vi "Actor Core.vi"(8 "error in":errorcluster, 11 "CS++OPCUAInterface in":refnum<class "CS++OPCUAInterface.lvclass">) -> (0 "error out":errorcluster, 3 "Actor out":refnum<class "Actor.lvclass">)   [LabVIEW 2015, in "CS++OPCUAInterface.lvlib" / "CS++OPCUAInterface.lvclass"]
doc: "Register OPCUA-Item vor values change events and write new data to PV-Read-URLs.\n\n\n(<B>Filename</B>: Actor Framework.lvlib:Actor.lvclass:Actor Core.vi)\n\nReceives messages to the actor, reacts to them, and initiates any error handling that may shut the actor down.\n\nDescendant classes may override this VI to append parallel tasks for the actor to complete while it handles messages. Overrides use the Call Parent Method node."
uses:
  CS++OPCUAInterface.lvclass
  <vilib>/ActorFramework/Actor/Actor.lvclass
  CS++OPCUAInterface.lvclass/CS++OPCUAInterface.ctl
  CSPP_Core/Actors/CS++BaseActor/CS++BaseActor.lvclass/CS++BaseActor.ctl
  CSPP_Core/Classes/CS++ProcessVariables/ProcessVariable/PV.lvclass
  CSPP_Core/Classes/CS++ProcessVariables/ProcessVariable/PV.lvclass/PV.ctl
  <vilib>/ActorFramework/Actor/Actor.lvclass/Actor.ctl
  <vilib>/ActorFramework/Message Enqueuer/Message Enqueuer.lvclass/Message Enqueuer.ctl
  <vilib>/ActorFramework/Report Error Msg/Report Error Msg.lvclass/Report Error Msg.ctl
  CSPP_Core/Classes/CS++ProcessVariables/ProcessVariable/Write Data.vi
  CSPP_Core/Classes/CS++ProcessVariables/ProcessVariable/Write Timestamp.vi
  CSPP_Core/Classes/CS++ProcessVariables/ProcessVariable/Write status.vi
  CSPP_Core/Classes/CS++ProcessVariables/ProcessVariable/Write Quality.vi
  CSPP_Core/Classes/CS++ProcessVariables/ProcessVariable/Write Error.vi
  CSPP_Core/Actors/CS++BaseActor/Read Polling Interval.vi
  <vilib>/ActorFramework/Message Enqueuer/Init from Existing Queue.vi
  <vilib>/ActorFramework/Message Enqueuer/Enqueue.vi
  <vilib>/ActorFramework/Message Priority Queue/Priority Enqueue.vi
  <vilib>/ActorFramework/Message Enqueuer/Message Enqueuer.lvclass
  <vilib>/ActorFramework/Report Error Msg/Report Error Msg.lvclass
  CSPP_Core/Actors/CS++BaseActor/CS++BaseActor.lvclass
  <vilib>/OPCUA/NI OPC UA Client.lvlib
  CSPP_Core/Classes/CS++ProcessVariables/PVConnection/PVConnection.lvclass
panel:
  out "Data":T1
  out "Size":i32
  out "OPCUA-Item":string
  out "PV-URL":string
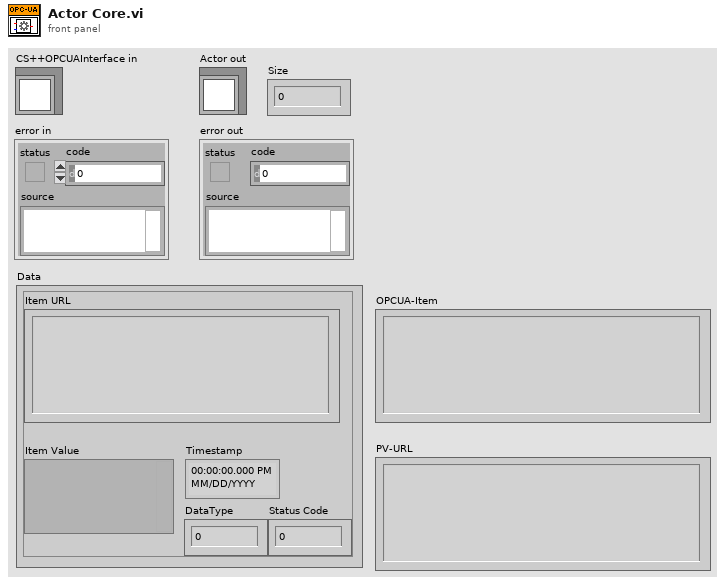
[diagram p1: front panel]
types:
  T1 = cluster{"Item URL":string, "Item Value":variant, "Timestamp":timestamp, "DataType":u32, "Status Code":u32}
  T2 = cluster{"queue size(1)":u32, "discard oldest(T)":bool}
  T3 = cluster{"Item URL":string, "Item Value":variant, "Timestamp":timestamp, "DataType":u32, "status code":u32}[]
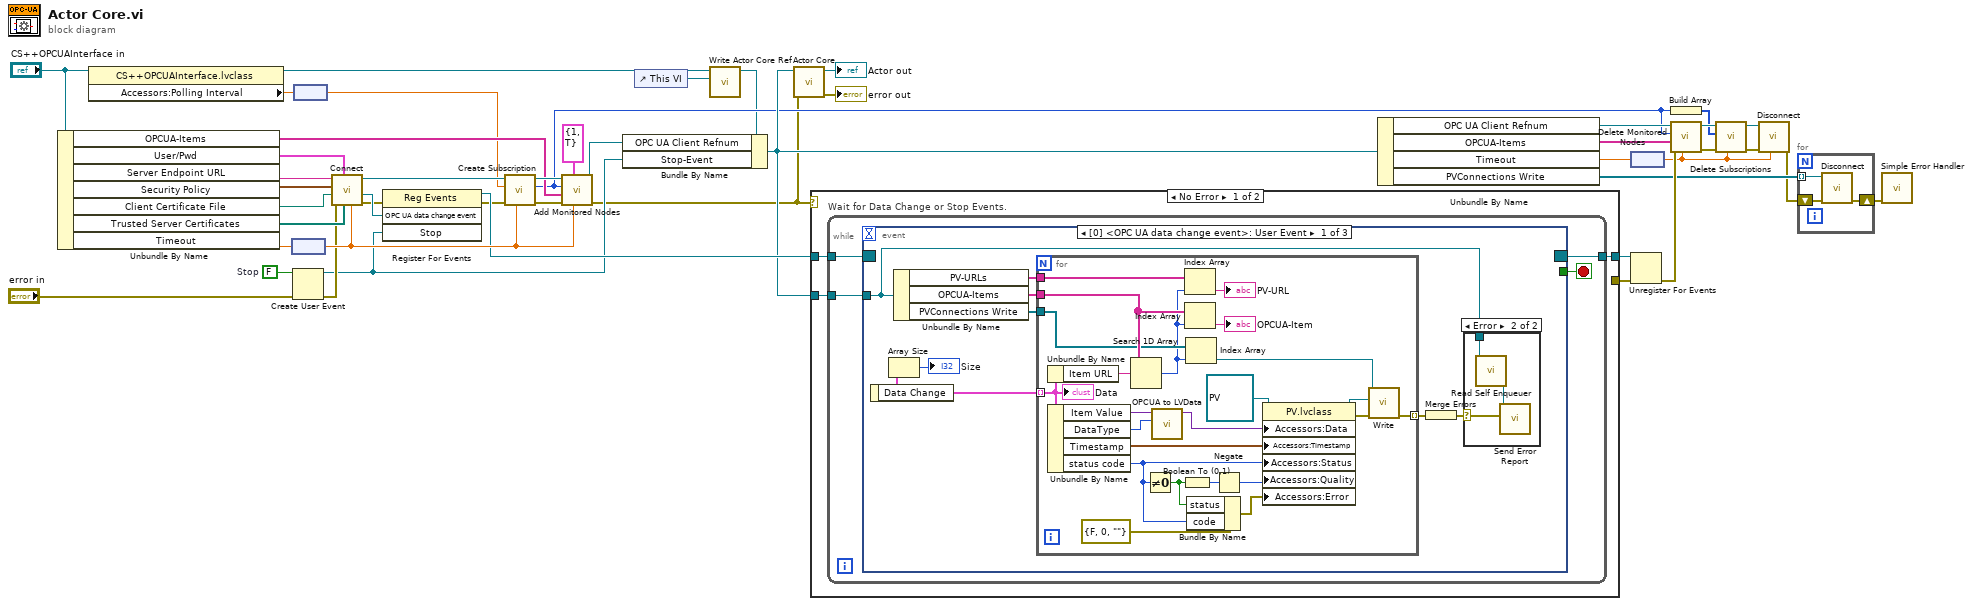
[diagram p0: block diagram]
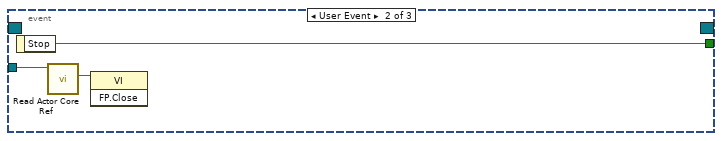
[diagram p3: hidden frame]
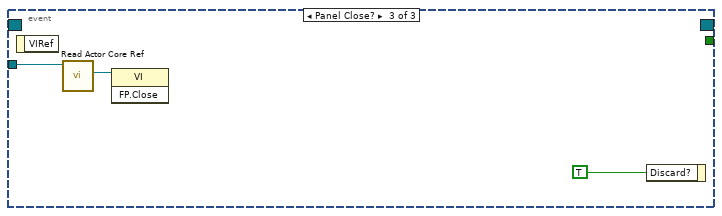
[diagram p4: hidden frame]
diagram:
  w28 = FALSE  # Stop
  n1 = Unbundle By Name("CS++OPCUAInterface in") -> ("OPCUA-Items"=w35:string[], "User/Pwd"=w44:cluster{"Username":string, "Password":string}, "Server Endpoint URL"=w45:string, "Security Policy"=w43:cluster{"Message Mode":u16, "Security":u16}, "Client Certificate File"=w42:path, "Trusted Server Certificates"=w41:path[], "Timeout"=w40:dbl[unit])
  n2 = property class="CS++OPCUAInterface.lvclass"(reference="CS++OPCUAInterface in") -> (reference out=w3:refnum<class "CS++OPCUAInterface.lvclass">, "Accessors:Polling Interval"=w9:dbl[unit])  [unwired: 1 in, 1 out]
  n3 = node(w40) -> (w34:dbl)
  n4 = Create User Event(user event datatype=w28, error in="error in") -> (user event=w25:refnum<user-event>, error out=w26:errorcluster)
  n5 = node(w9) -> (w31:dbl)
  n6 = call <vilib>:"Connect.vi"("timeout (5000 ms)"=w34, "trusted server certificates"=w41, "username/password"=w44, "error in (no error)"=w26, "client certificate file"=w42, "security policy"=w43, "server endpoint URL"=w45) -> ("error out"=w30:errorcluster, "OPC UA data change event"=w39:refnum<user-event>, "OPC UA client refnum out"=w38:refnum<k21>)  [unwired: 2 in]
  n7 = register-events(error in=w30, w39, w25) -> (reference out=w32:refnum<event-registration>, error out=w29:errorcluster)  [unwired: 1 in]
  n8 = call <vilib>:"Create Subscription.vi"("timeout (5000 ms)"=w34, "error in (no error)"=w29, "update rate (1000 ms)"=w31, "OPC UA client refnum in"=w38) -> ("error out"=w36:errorcluster, "subscription ID out"=w17:u32, "OPC UA client refnum out"=w37:refnum<k21>)  [unwired: 5 in]
  n9 = call <vilib>:"Add Monitored Nodes.vi"("timeout (5000 ms)"=w34, "notification queue settings"=T2 {"queue size(1)"=1, "discard oldest(T)"=TRUE}, "error in (no error)"=w36, "array of node path"=w35, "subscription ID in"=w17, "OPC UA client refnum in"=w37) -> ("error out"=w8:errorcluster, "OPC UA client refnum out"=w33:refnum<k21>)  [unwired: 3 in, 1 out]
  n10 = control-ref of="This VI"() -> (w1:refnum<vi>)
  n11 = call "Write Actor Core Ref.vi"("Actor Core Ref"=w1, "CS++BaseActor in"=w3) -> ("CS++BaseActor out"=w2:refnum<class "CS++OPCUAInterface.lvclass">)  [unwired: 8 in, 1 out]
  n12 = Bundle By Name(cluster=w2, "OPC UA Client Refnum"=w33, "Stop-Event"=w25) -> (w20:refnum<class "CS++OPCUAInterface.lvclass">)
  n13 = call-parent "Actor Core.vi"("error in"=w8, "CS++BaseActor in"=w20) -> ("error out"=→"error out":errorcluster, "Actor out"=→"Actor out":refnum<class "Actor.lvclass">)  [unwired: 8 in]
  n14 = case shown="No Error" w8 {
    selector: w8 -> [_ w95]
    tunnel: w32 -> [w50 w96]
    tunnel: [w49 w96] -> w24
    tunnel: w20 -> [w48 _]
    tunnel: [_ w95] -> w7
    frame No Error {
      n15 = while "Wait for Data Change or Stop Events." {
        tunnel: w50 -> [w54]
        tunnel: w48 -> [w51]
        tunnel: [w52] -> w49
        stop <- w53 stop-if-true
        n16 = event shown="[0] <OPC UA data change event>: User Event" {
          selector: w54 -> [_ _ _]
          dyn-events: [_ _ _] -> w52
          timeout: _ -> [_ _ _]
          tunnel: [_ w91 _] -> w53
          tunnel: w51 -> [w56 w90 w92]
          event User Event {
            n17 = event-data() -> ("Data Change"=w59:T3)  [unwired: 1 in]
            n18 = Array Size(array=w59) -> (size(s)=→"Size":i32)
            n19 = Unbundle By Name(w56) -> ("PV-URLs"=w62:string[], "OPCUA-Items"=w61:string[], "PVConnections Write"=w58:refnum<class "PVConnection.lvclass">[])
            n20 = for {
              tunnel: w62 -> [w88]
              tunnel: w61 -> [w85]
              tunnel: w59 -> [w81] mode=indexing
              tunnel: w58 -> [w83]
              tunnel: [w71] -> w57 mode=indexing
              n21 = Unbundle By Name(w81) -> ("Item URL"=w84:string)
              n22 = Unbundle By Name(w81) -> ("Item Value"=w68:variant, "DataType"=w66:u32, "Timestamp"=w80:timestamp, "status code"=w75:u32)
              n23 = Search 1D Array(1D array=w85, element=w84) -> (index of element=w82:i32)  [unwired: 1 in]
              n24 = Not Equal To 0?(x=w75) -> (x != 0?=w74:bool)
              n25 = call "OPCUA to LVData.vi"("DataType"=w66, "OPCUA Variant in"=w68) -> ("OPCUA Variant out"=w67:variant)  [unwired: 8 in, 1 out]
              n26 = Boolean To (0,1)(Boolean=w74) -> (0, 1=w79:i16)
              n27 = Index Array(array=w88, index=w82) -> (element=→"PV-URL":string)
              n28 = Index Array(array=w85, index=w82) -> (element=→"OPCUA-Item":string)
              n29 = Index Array(array=w83, index=w82) -> (element=w69:refnum<class "PVConnection.lvclass">)
              n30 = Bundle By Name(cluster=errorcluster {"status"=FALSE, "code"=0, "source"=""} ("Error"), "status"=w74, "code"=w75) -> (w76:errorcluster)
              n31 = Negate(x=w79) -> (-x=w78:i16)
              n32 = property class="PV.lvclass"(reference=refnum<class "PV.lvclass"> refnum ("CS++ProcessVariables.lvlib:PV.lvclass"), "Accessors:Data"=w67, "Accessors:Timestamp"=w80, "Accessors:Status"=w75, "Accessors:Quality"=w78, "Accessors:Error"=w76) -> (reference out=w73:refnum<class "PV.lvclass">, error out=w72:errorcluster)  [unwired: 1 in]
              n33 = call "Write.vi"("error in (no error)"=w72, "PV"=w73, "PVConnection in"=w69) -> ("error out"=w71:errorcluster)  [unwired: 7 in, 1 out]
              "Data" <- w81
            }
            n34 = Merge Errors(w57) -> (w55:errorcluster)
            n35 = case shown="Error" w55 {
              selector: w55 -> [_ w63]
              tunnel: w56 -> [_ w65]
              frame No Error {
              }
              frame Error {
                n36 = call <vilib>:"Read Self Enqueuer.vi"("Actor"=w65) -> ("Self Enqueuer"=w64:refnum<class "Message Enqueuer.lvclass">)  [unwired: 10 in]
                n37 = call <vilib>:"Send Error Report.vi"("Error From Sender"=w63, "Message Enqueuer"=w64) -> ()  [unwired: 9 in, 1 out]
              }
            }
          }
          event User Event {
            n38 = event-data() -> ("Stop"=w91:bool)  [unwired: 1 in]
            n39 = call "Read Actor Core Ref.vi"("CS++BaseActor in"=w90) -> ("Actor Core Ref"=w89:refnum<vi>)  [unwired: 8 in, 2 out]
            n40 = invoke class="VI" method="FP.Close"(reference=w89) -> ()  [unwired: 2 in, 3 out]
          }
          event Panel Close? {
            n41 = event-data() -> ()  [unwired: 1 in, 1 out]
            n42 = call "Read Actor Core Ref.vi"("CS++BaseActor in"=w92) -> ("Actor Core Ref"=w93:refnum<vi>)  [unwired: 8 in, 2 out]
            n43 = invoke class="VI" method="FP.Close"(reference=w93) -> ()  [unwired: 2 in, 3 out]
            n44 = event-data("Discard?"=TRUE) -> ()  [unwired: 1 in, 1 out]
          }
        }
      }
    }
    frame Error {
    }
  }
  n45 = Unbundle By Name(w20) -> ("OPC UA Client Refnum"=w18:refnum<k21>, "OPCUA-Items"=w19:string[], "Timeout"=w15:dbl[unit], "PVConnections Write"=w6:refnum<class "PVConnection.lvclass">[])
  n46 = node(w15) -> (w12:dbl)
  n47 = Unregister For Events(event registration refnum=w24, error in=w7) -> (error out=w22:errorcluster)
  n48 = Build Array(w17) -> (w16:u32[])
  n49 = call <vilib>:"Delete Monitored Nodes.vi"("timeout (5000 ms)"=w12, "error in (no error)"=w22, "array of node path"=w19, "subscription ID in"=w17, "OPC UA client refnum in"=w18) -> ("error out"=w21:errorcluster, "OPC UA client refnum out"=w23:refnum<k21>)  [unwired: 3 in, 2 out]
  n50 = call <vilib>:"Delete Subscriptions.vi"("timeout (5000 ms)"=w12, "error in (no error)"=w21, "array of subscription ID"=w16, "OPC UA client refnum in"=w23) -> ("error out"=w14:errorcluster, "OPC UA client refnum out"=w13:refnum<k21>)  [unwired: 5 in, 1 out]
  n51 = call <vilib>:"Disconnect.vi"("timeout (5000 ms)"=w12, "error in (no error)"=w14, "OPC UA client refnum in"=w13) -> ("error out"=w5:errorcluster)  [unwired: 8 in]
  n52 = for {
    tunnel: w6 -> [w99] mode=indexing
    shift-right: [w97] -> w4
    shift-left: w5 -> [w98]
    n53 = call <vilib>:"Disconnect.vi"("error in (no error)"=w98, "PVConnection in"=w99) -> ("error out"=w97:errorcluster)  [unwired: 8 in, 1 out]
  }
  n54 = call <vilib>:"Simple Error Handler.vi"("error in (no error)"=w4) -> ()  [unwired: 4 in, 5 out]
